vi "Run.vi"(8 "error in (no error)":errorcluster, 10 "Address":dbl=1.0, 11 "VISA resource name (IN)":refnum<visa-resource-name>) -> (0 "error out":errorcluster, 3 "VISA resource name (OUT)":refnum<visa-resource-name>)   [LabVIEW 2010, in "Yudian AI508.lvlib"]
uses:
  <instrlib>/Yudian AI508/Yudian AI508.lvlib
panel:
  out "Recieved Raw Data":string
  out "Recevied Temp.  data":dbl
  out "Data buffer":string
  out "Digital shift":i32
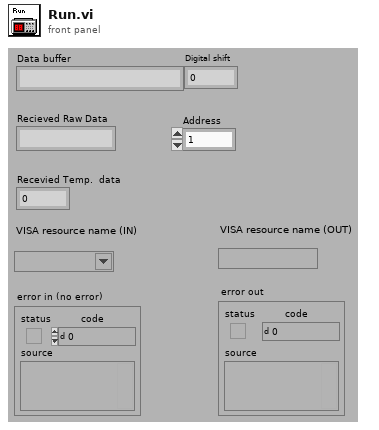
[diagram p1: front panel]
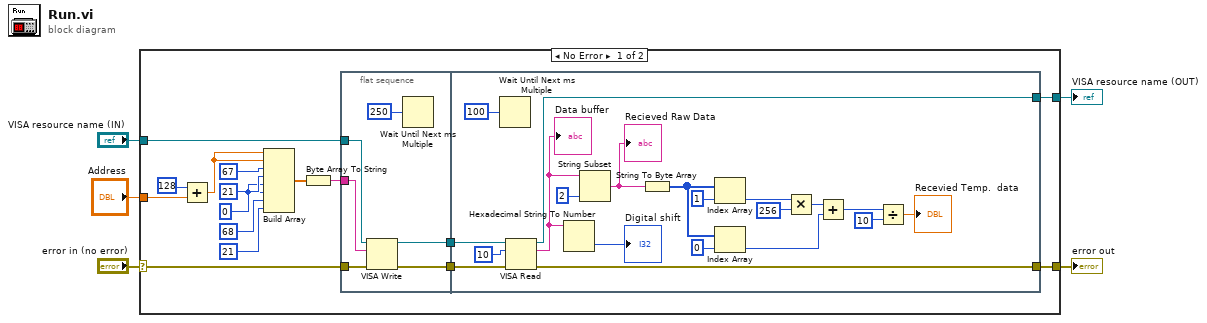
[diagram p0: block diagram]
diagram:
  n1 = case shown="No Error" "error in (no error)" {
    selector: "error in (no error)" -> [w16 w49]
    tunnel: [w18 w49] -> w5
    tunnel: [w19 w48] -> w4
    tunnel: "VISA resource name (IN)" -> [w17 w48]
    tunnel: "Address" -> [w9 _]
    frame No Error {
      w6 = 0
      n2 = Add(x=128, y=w9) -> (x+y=w7:dbl)
      n3 = Build Array(w7, w7, 67, 21, w6, w6, 68, 21) -> (w11:dbl[])
      n4 = Byte Array To String(unsigned byte array=w11) -> (string=w10:string)
      n5 = flat-sequence {
        tunnel: w16 -> [w27]
        tunnel: w17 -> [w24]
        tunnel: [w26] -> w21
        tunnel: [w25] -> w20
        tunnel: w10 -> [w22]
        tunnel: w21 -> [w33]
        tunnel: w20 -> [w32]
        tunnel: [w30] -> w19
        tunnel: [w29] -> w18
        frame #0 {
          n6 = VISA Write(VISA resource name=w24, write buffer=w22, error in (no error)=w27) -> (VISA resource name out=w25:refnum<visa-resource-name>, error out=w26:errorcluster)  [unwired: 1 out]
          n7 = Wait Until Next ms Multiple(millisecond multiple=250) -> ()  [unwired: 1 out]
        }
        frame #1 {
          n8 = Wait Until Next ms Multiple(millisecond multiple=100) -> ()  [unwired: 1 out]
          n9 = VISA Read(VISA resource name=w32, byte count=u32 10 ("字节总数"), error in (no error)=w33) -> (VISA resource name out=w30:refnum<visa-resource-name>, read buffer=w35:string, error out=w29:errorcluster)  [unwired: 1 out]
          "Data buffer" <- w35
          n10 = Hexadecimal String To Number(string=w35) -> (number=→"Digital shift":u32)  [unwired: 3 out]
          n11 = String Subset(string=w35, length (rest)=2 ("length (rest)")) -> (substring=w45:string)  [unwired: 1 out]
          "Recieved Raw Data" <- w45
          n12 = String To Byte Array(string=w45) -> (unsigned byte array=w43:u8[])
          n13 = Index Array(array=w43, index=1) -> (element=w42:u8)
          n14 = Index Array(array=w43, index=0) -> (element=w39:u8)
          n15 = Multiply(x=w42, y=u16 256) -> (x*y=w40:u16)
          n16 = Add(x=w40, y=w39) -> (x+y=w38:u16)
          n17 = Divide(x=w38, y=u16 10) -> (x/y=→"Recevied Temp.  data":dbl)
        }
      }
    }
    frame Error {
    }
  }
  "error out" <- w5
  "VISA resource name (OUT)" <- w4
